vi "Single Z Ramp Approach Descriptor.vi"() -> (0 "Experimental Data Save VI Reference":refnum<vi>, 1 "Experimental VI Reference":refnum<vi>, 2 "Experimental VI Icon":picture, 3 "Experimental VI Description":string)   [LabVIEW 2013]
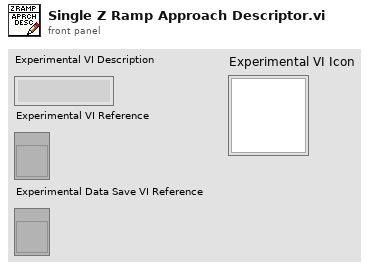
[diagram p1: front panel]
types:
  T1 = typedef "imagedata.ctl" = cluster{"image type":i32, "image depth":i32, "image":u8[], "mask":u8[], "colors":u32[], "Rectangle":cluster{"left":i16, "top":i16, "right":i16, "bottom":i16}}
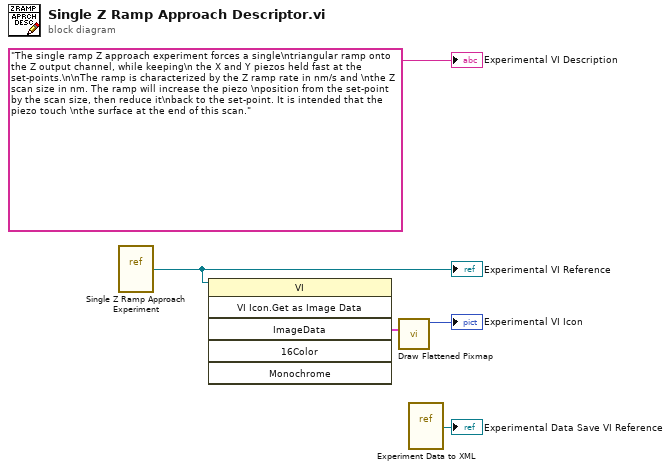
[diagram p0: block diagram]
diagram:
  n1 = vi-ref "Single Z Ramp Approach Experiment.vi"() -> (w2:refnum<vi>)
  "Experimental VI Reference" <- w2
  n2 = invoke class="VI" method="VI Icon.Get as Image Data"(reference=w2) -> ("ImageData"=w3:T1)  [unwired: 5 in, 5 out]
  n3 = call <vilib>:"Draw Flattened Pixmap.vi"("image data"=w3) -> ("new picture"=→"Experimental VI Icon":picture)  [unwired: 8 in]
  n4 = vi-ref "Experiment Data to XML.vi"() -> (→"Experimental Data Save VI Reference":refnum<vi>)
  "Experimental VI Description" <- "The single ramp Z approach experiment forces a single\ntriangular ramp onto the Z output channel, while keeping\n the X and Y piezos held fast at the set-points.\n\nThe ramp is characterized by the Z ramp rate in nm/s and \nthe Z scan size in nm. The ramp will increase the piezo \nposition from the set-point by the scan size, then reduce it\nback to the set-point. It is intended that the piezo touch \nthe surface at the end of this scan."
